vi "CAN_TEST.vi"() -> ()   [LabVIEW 2019]
uses:
  Libraries/ZLG_CAN/ZLG_CAN.lvlib
panel:
  in  "START":bool
  out "数组":string[](array[string])
  in  "帧数据":T1={"[0]"=3, "[1]"=34, "[2]"=241, "[3]"=148, "[4]"=0, "[5]"=0, "[6]"=0, "[7]"=0} {"[0]" format="%x"; "[1]" format="%x"; "[2]" format="%x"; "[3]" format="%x"; "[4]" format="%x"; "[5]" format="%x"; "[6]" format="%x"; "[7]" format="%x"}
  in  "帧格式":enum16{"数据帧", "远程帧"}(ring)
  in  "帧类型":enum8{"标准帧", "扩展帧"}(ring)
  in  "ID":u32=1828 format="0x%x"
  in  "波特率":u32(ring)=11 items=["5Kbps", "10Kbps", "20Kbps", "40Kbps", "50Kbps", "80Kbps", "100Kbps", "125Kbps", "200Kbps", "250Kbps", "400Kbps", "500Kbps", "666Kbps", "800Kbps", "1000Kbps"]
  in  "CAN 通道":u32(ring) items=["0", "1"]
  in  "索引":u32(ring) items=["0", "1", "2", "3", "4", "5", "6", "7", "8"]
  in  "设备类型":u32(ring)=27 items=["PCI5121"=1, "PCI9810"=2, "USBCAN1"=3, "USBCAN2"=4, "PCI9820"=5, "PCI5110"=7, "PC104CAN"=11, "CANETUDP"=12, "PCI9840B"=14, "PC104C2"=15, "PCI9820I"=16, "CANETTCP"=17, "PCIE9221"=24, "PCI5010U"=19, "USBCAN_E_U"=20, "USBCAN_2E_U"=21, "PCI5020U"=22, "PCIE9120I"=27, "PCIE9110I"=28, "PCIE9140I"=29]
  in  "Stop":bool
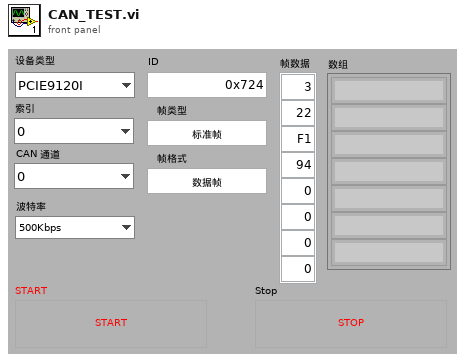
[diagram p1: front panel]
types:
  T1 = cluster{"[0]":u8, "[1]":u8, "[2]":u8, "[3]":u8, "[4]":u8, "[5]":u8, "[6]":u8, "[7]":u8}
  T2 = typedef "ZLG_CAN.lvlib/Start_CAN (Reply Payload)--cluster.ctl" = cluster{"Success":bool, "Start_CAN_error":errorcluster}
  T3 = typedef "ZLG_CAN.lvlib/Sent_Recive (Reply Payload)--cluster.ctl" = cluster{"Receive":T4[], "Sent_Recive_error":errorcluster}
  T4 = typedef "ZLG_CAN.lvlib/CAN_OBJ_R.ctl" = cluster{"ID":u32, "TimeStamp":u32, "TimeFlag":u8, "SendType":u8, "RemoteFlag":u8, "ExternFlag":u8, "DataLen":u8, "数值":u8, "数值":u8, "数值":u8, "数值":u8, "数值":u8, "数值":u8, "数值":u8, "数值":u8, "数值":u8, "数值":u8, "数值":u8}
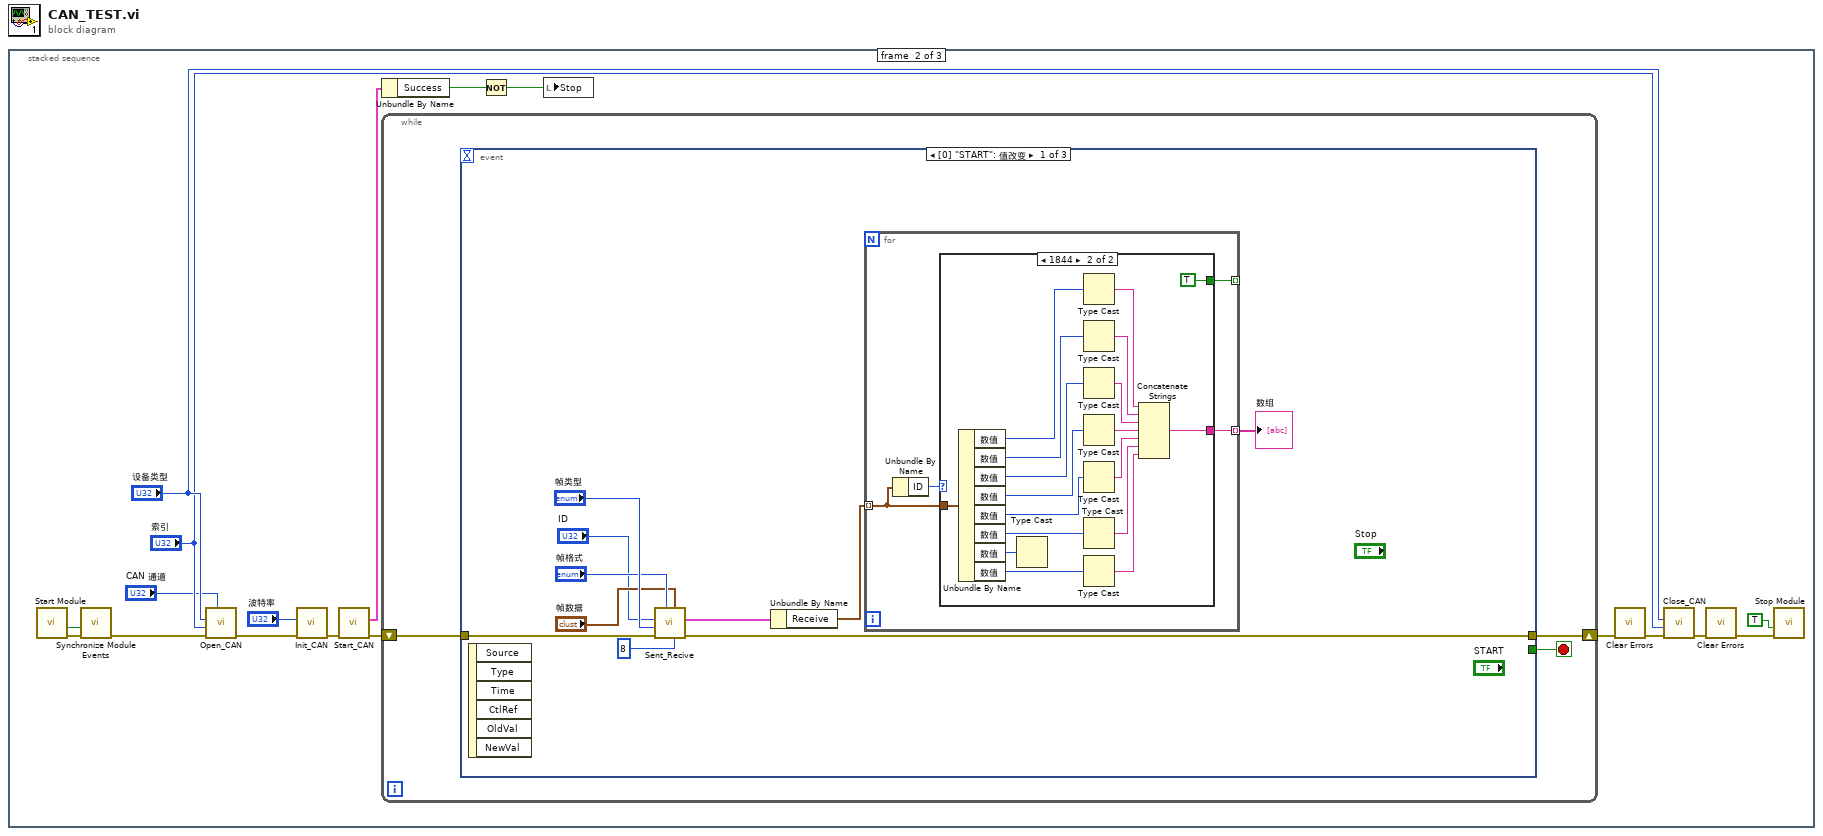
[diagram p0: block diagram]
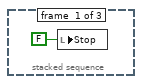
[diagram p2: hidden frame]
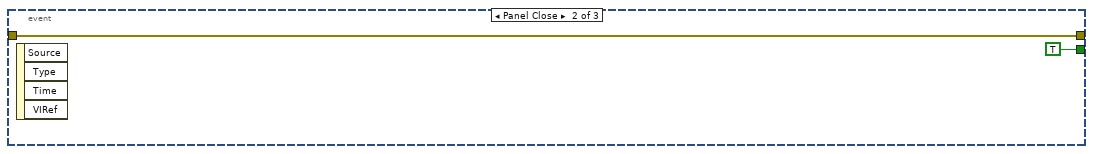
[diagram p4: hidden frame]
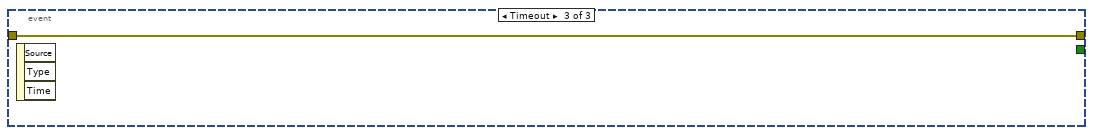
[diagram p5: hidden frame]
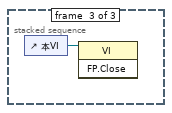
[diagram p6: hidden frame]
diagram:
  n1 = stacked-sequence {
    frame #0 {
      n2 = local write "Stop"(FALSE ("Stop")) -> ()
    }
    frame #1 {
      n3 = call "Start Module.vi"() -> ("error out"=w19:errorcluster, "Wait for Event Sync?"=w18:bool)  [unwired: 8 in, 2 out]
      n4 = call "Synchronize Module Events.vi"("error in (no error)"=w19, "Wait for Event Sync?"=w18) -> ("error out"=w17:errorcluster)  [unwired: 9 in]
      n5 = call "Open_CAN.vi"("CAN 通道"="CAN 通道", "error in (no error)"=w17, "索引"="索引", "设备类型"="设备类型") -> ("error out"=w14:errorcluster)  [unwired: 7 in]
      n6 = call "Init_CAN.vi"("error in (no error)"=w14, "波特率"="波特率") -> ("error out"=w10:errorcluster)  [unwired: 9 in]
      n7 = call "Start_CAN.vi"("error in (no error)"=w10) -> ("error out"=w5:errorcluster, "Reply Payload"=w12:T2)  [unwired: 8 in, 1 out]
      n8 = Unbundle By Name(w12) -> ("Success"=w11:bool)
      n9 = while {
        shift-right: [w21] -> w2
        shift-left: w5 -> [w22]
        stop <- w20 stop-if-true
        n10 = event shown="[0] \"START\": 值改变" {
          selector: _ -> [_ _ _]
          dyn-events: _ -> [_ _ _]
          timeout: _ -> [_ _ _]
          tunnel: w22 -> [w25 w55 w57]
          tunnel: [w24 w55 w57] -> w21
          tunnel: [_ TRUE _] -> w20
          event "START": Value Change {
            n11 = event-data() -> ()  [unwired: 1 in, 6 out]
            n12 = call "Sent_Recive.vi"("帧长度"=u8 8, "CAN_FRAME"="帧数据", "帧格式"="帧格式", "error in (no error)"=w25, "帧类型"="帧类型", "ID"="ID") -> ("error out"=w24:errorcluster, "Reply Payload"=w23:T3)  [unwired: 3 in, 1 out]
            n13 = Unbundle By Name(w23) -> ("Receive"=w32:T4[])
            n14 = for {
              tunnel: w32 -> [w35] mode=indexing
              tunnel: [w34] -> w31 mode=indexing
              tunnel: [w33] -> _ mode=indexing
              n15 = Unbundle By Name(w35) -> ("ID"=w36:u32)
              n16 = case shown="1844" w36 {
                tunnel: w35 -> [_ w54]
                tunnel: [_ w38] -> w34
                tunnel: [_ TRUE] -> w33
                frame 0, Default {
                }
                frame 1844 {
                  n17 = Unbundle By Name(w54) -> ("数值"=w53:u8, "数值"=w52:u8, "数值"=w51:u8, "数值"=w50:u8, "数值"=w49:u8, "数值"=w48:u8, "数值"=w47:u8, "数值"=w46:u8)
                  n18 = Type Cast(x=w47) -> ()  [unwired: 1 in, 1 out]
                  n19 = Type Cast(x=w53) -> (*(type *) &x=w45:string)  [unwired: 1 in]
                  n20 = Type Cast(x=w52) -> (*(type *) &x=w44:string)  [unwired: 1 in]
                  n21 = Type Cast(x=w51) -> (*(type *) &x=w43:string)  [unwired: 1 in]
                  n22 = Type Cast(x=w50) -> (*(type *) &x=w42:string)  [unwired: 1 in]
                  n23 = Type Cast(x=w49) -> (*(type *) &x=w41:string)  [unwired: 1 in]
                  n24 = Type Cast(x=w48) -> (*(type *) &x=w40:string)  [unwired: 1 in]
                  n25 = Type Cast(x=w46) -> (*(type *) &x=w39:string)  [unwired: 1 in]
                  n26 = Concatenate Strings(w45, w44, w43, w42, w41, w40, w39) -> (w38:string)
                }
              }
            }
            "数组" <- w31
          }
          event Panel Close {
            n27 = event-data() -> ()  [unwired: 1 in, 4 out]
          }
          event Timeout {
            n28 = event-data() -> ()  [unwired: 1 in, 3 out]
          }
        }
      }
      n29 = Not(x=w11) -> (.not. x?=w4:bool)
      n30 = local write "Stop"(w4) -> ()
      n31 = call <vilib>:"Clear Errors.vi"("error in (no error)"=w2) -> ("error out"=w6:errorcluster)  [unwired: 5 in, 1 out]
      n32 = call "Close_CAN.vi"("error in (no error)"=w6, "索引"="索引", "设备类型"="设备类型") -> ("error out"=w9:errorcluster)  [unwired: 8 in]
      n33 = call <vilib>:"Clear Errors.vi"("error in (no error)"=w9) -> ("error out"=w7:errorcluster)  [unwired: 5 in, 1 out]
      n34 = call "Stop Module.vi"("error in (no error)"=w7, "Wait for Module to Stop? (F)"=TRUE) -> ()  [unwired: 9 in, 1 out]
    }
    frame #2 {
      n35 = control-ref of="本VI"() -> (w58:refnum<vi>)
      n36 = invoke class="VI" method="FP.Close"(reference=w58) -> ()  [unwired: 2 in, 3 out]
    }
  }
